vi "Calcualte N_total and Updates.vi"(2 "Sampling":cluster{"Fs":dbl, "#s":i32}, 3 "Sweep Time (s)":dbl) -> (0 "Updates":i32, 1 "N_Total":i32)   [LabVIEW 2019, in "Instrument.DAQ.lvclass"]
uses:
  Instrument.DAQ.lvclass
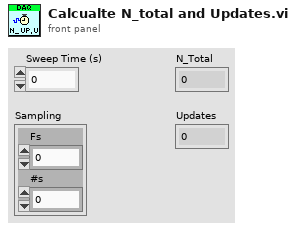
[diagram p1: front panel]
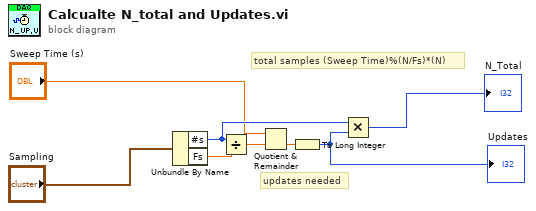
[diagram p0: block diagram]
diagram:
  # "updates needed"
  # "total samples (Sweep Time)%(N/Fs)*(N)"
  n1 = Unbundle By Name("Sampling") -> ("#s"=w6:i32, "Fs"=w5:dbl)
  n2 = Divide(x=w6, y=w5) -> (x/y=w3:dbl)
  n3 = Quotient & Remainder(x="Sweep Time (s)", y=w3) -> (floor(x/y)=w4:dbl)  [unwired: 1 out]
  n4 = To Long Integer(number=w4) -> (32bit integer=w7:i32)
  "Updates" <- w7
  n5 = Multiply(x=w6, y=w7) -> (x*y=→"N_Total":i32)
